vi "testVisionWebService.vi"() -> ()   [LabVIEW 2017]
uses:
  DataAccessors/action.ctl
  DataAccessors/VisionWebServiceData.lvlib
  DataAccessors/message.ctl
  cRIO/Thermography/RT/subVIs/Utility/DetectCameras/CameraInfo.ctl
  cRIO/Thermography/RT/subVIs/Acquisition/controls/imagePalette.ctl
  cRIO/Thermography/RT/subVIs/Acquisition/controls/imageDisaplyInfo.ctl
panel:
  in  "Tab Control":enum32{"CameraInfo", "DisplayConfig", "Image"}(tab)
  in  "CameraInfo":T1[](array[typedef])=[{"InterfaceName"="cam0", "VendorName"="FLIR", "ModelName"="Ax5", "CameraFileName"="test", "SerialNumber"="123d465", "IP Address"="10.2.43.65", "PhysicalPort"="1", "CameraName"=""}]
  in  "display cfg":T2[](array[typedef])=[{"cameraSerialNumber"="12344", "autoscale"=TRUE, "userMin"=-12.0, "userMax"=56.0, "palette"={"currentValue"="rainbow", "possibleValues"=["normal"]}}]
  in  "File Path":path
  in  "Stop Button":bool
  out "IterationCount":i32=985
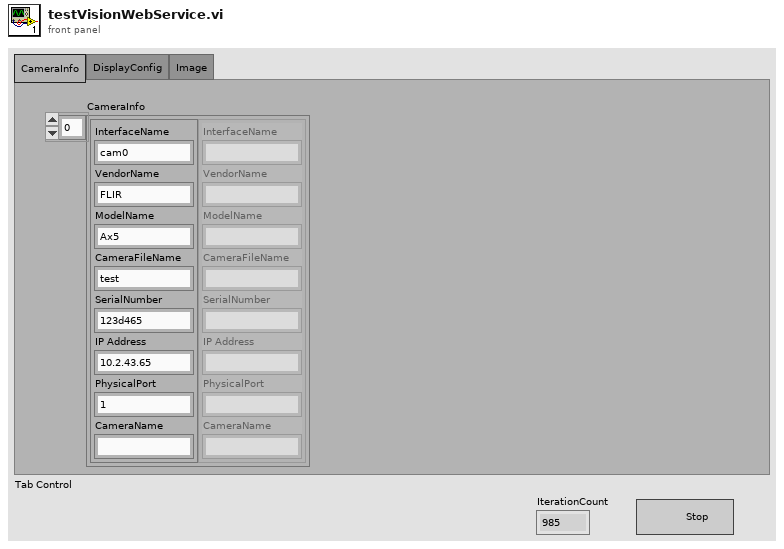
[diagram p1: front panel]
types:
  T1 = typedef "CameraInfo.ctl" = cluster{"InterfaceName":string, "VendorName":string, "ModelName":string, "CameraFileName":string, "SerialNumber":string, "IP Address":string, "PhysicalPort":string, "CameraName":string}
  T2 = typedef "IR_Acquisition.lvlib/imageDisaplyInfo.ctl" = cluster{"cameraSerialNumber":string, "autoscale":bool, "userMin":dbl, "userMax":dbl, "palette":T3}
  T3 = typedef "IR_Acquisition.lvlib/imagePalette.ctl" = cluster{"currentValue":string, "possibleValues":string[]}
  T4 = typedef "VisionWebServiceData.lvlib/action.ctl" = enum16{"Get", "Set"}
  T5 = typedef "VisionWebServiceData.lvlib/message.ctl" = cluster{"name":string, "value":string}
  T6 = typedef "Image Type" = u32
  T7 = typedef "IMAQ Image.ctl" = refnum<image>
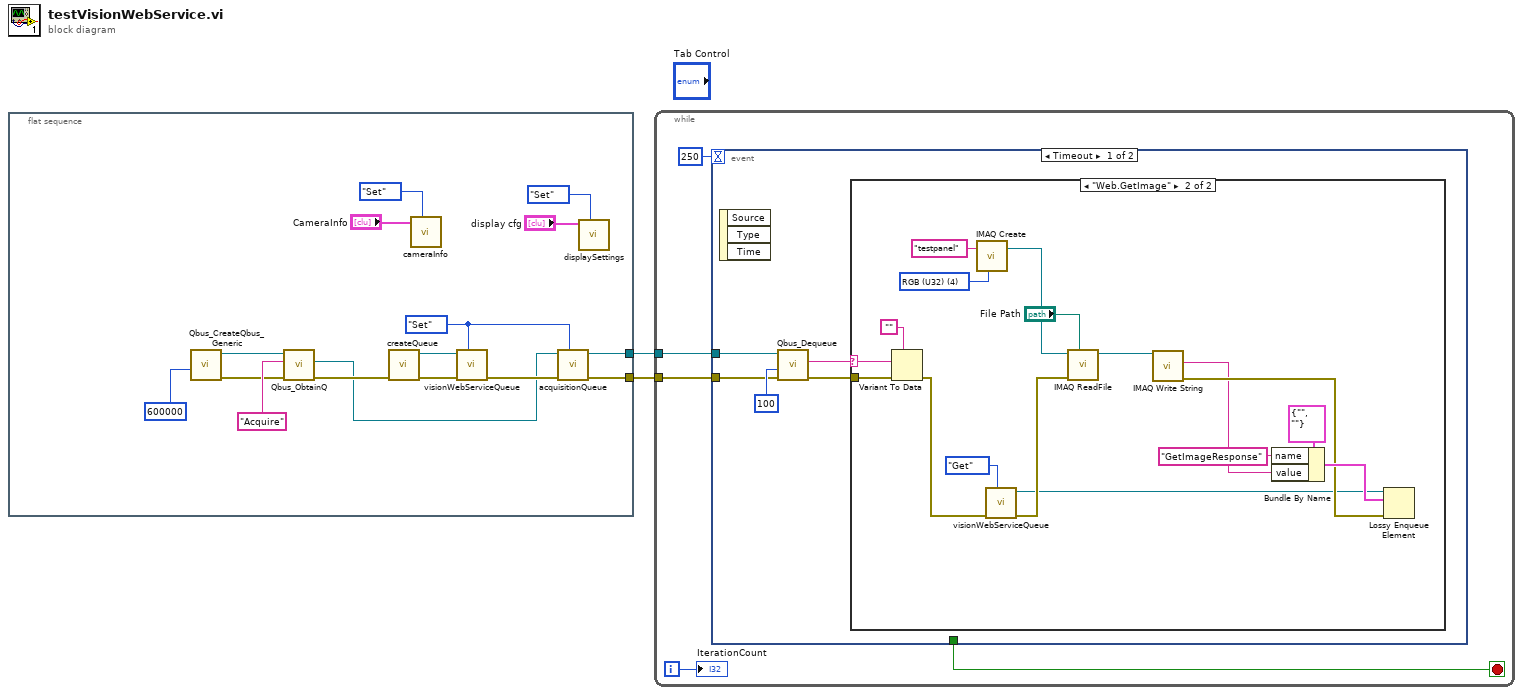
[diagram p0: block diagram]
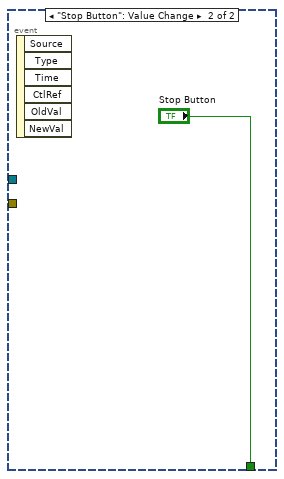
[diagram p3: hidden frame]
diagram:
  n1 = flat-sequence {
    tunnel: [w14] -> w2
    tunnel: [w6] -> w1
    frame #0 {
      w15 = action."Set" ("action")
      n2 = call <vilib>:"Qbus_CreateQbus_Generic.vi"("Timeout"=u32 600000) -> ("error out"=w4:errorcluster, "Qbus out"=w3:refnum<data-value>)  [unwired: 9 in]
      n3 = call <vilib>:"Qbus_ObtainQ.vi"("error in (no error)"=w4, "Qname"="Acquire", "Qbus in"=w3) -> ("error out"=w8:errorcluster, "Q out"=w7:refnum<data-value>)  [unwired: 5 in, 2 out]
      n4 = call "createQueue.vi"("error in (no error)"=w8) -> ("error out"=w18:errorcluster, "queue out"=w17:refnum<queue>)  [unwired: 9 in]
      n5 = call "cameraInfo.vi"("action"=action."Set", "CameraInfo"="CameraInfo") -> ()  [unwired: 8 in, 2 out]
      n6 = call "visionWebServiceQueue.vi"("action"=w15, "error in (no error)"=w18, "queue"=w17) -> ("error out"=w16:errorcluster)  [unwired: 7 in, 1 out]
      n7 = call "acquisitionQueue.vi"("action"=w15, "error in (no error)"=w16, "queue"=w7) -> ("error out"=w14:errorcluster, "queue"=w6:refnum<data-value>)  [unwired: 7 in]
      n8 = call "displaySettings.vi"("action"=action."Set", "display cfg"="display cfg") -> ()  [unwired: 8 in, 2 out]
    }
  }
  n9 = while {
    tunnel: w2 -> [w20]
    tunnel: w1 -> [w19]
    i -> [w21]
    stop <- w22 stop-if-true
    n10 = event shown="[0] Timeout" {
      selector: _ -> [_ _]
      dyn-events: _ -> [_ _]
      timeout: 250 -> [_ _]
      tunnel: [_ "Stop Button"] -> w22
      tunnel: w20 -> [w26 _]
      tunnel: w19 -> [w27 _]
      event Timeout {
        n11 = event-data() -> ()  [unwired: 1 in, 3 out]
        n12 = call <vilib>:"Qbus_Dequeue.vi"("error in (no error)"=w26, "timeout (0)"=100 ("milliseconds to wait"), "Q in"=w27) -> ("error out"=w24:errorcluster, "MsgName"=w25:string)  [unwired: 2 in, 5 out]
        n13 = case shown="\"Web.GetImage\"" w25 {
          selector: w25 -> [_ w42]
          tunnel: w24 -> [_ w41]
          frame "False", Default {
          }
          frame "Web.GetImage" {
            w33 = T6 4 items=["Grayscale (U8)", "Grayscale (I16)", "Grayscale (SGL)", "Complex (CSG)", "RGB (U32)", "HSL (U32)", "RGB (U64)", "Grayscale (U16)"] ("Image Type")
            n14 = Variant To Data(error in=w41, type="", Variant=w42) -> (error out=w44:errorcluster)  [unwired: 1 out]
            n15 = call "IMAQ Create"("Image Name"="testpanel", "Image Type"=w33) -> ("New Image"=w32:T7)  [unwired: 3 in, 1 out]
            n16 = call "visionWebServiceQueue.vi"("action"=action."Get", "error in (no error)"=w44) -> ("error out"=w35:errorcluster, "queue out"=w29:refnum<queue>)  [unwired: 8 in]
            n17 = call "IMAQ ReadFile"("File Path"="File Path", "error in (no error)"=w35, "Image"=w32) -> ("Image Out"=w34:T7)  [unwired: 4 in, 4 out]
            n18 = call-poly "IMAQ Write String"("Image"=w34) -> ("error out"=w37:errorcluster, "FileString"=w36:string)  [unwired: 8 in, 1 out]
            n19 = Bundle By Name(cluster=T5 {"name"="", "value"=""} ("element"), "name"="GetImageResponse", "value"=w36) -> (w39:T5)
            n20 = Lossy Enqueue Element(queue=w29, element=w39, error in (no error)=w37) -> ()  [unwired: 4 out]
          }
        }
      }
      event "Stop Button": Value Change {
        n21 = event-data() -> ()  [unwired: 1 in, 6 out]
      }
    }
    "IterationCount" <- w21
  }
